vi "Log to Excel.vi"(8 "error in":errorcluster, 11 "tdms file in":refnum<k34>) -> (0 "error out":errorcluster, 2 "appended array":dbl[][][](array[numeric]), 3 "tdms file out":refnum<k34>)   [LabVIEW 2014, in "Logger.lvlib"]
uses:
  Logger.lvlib
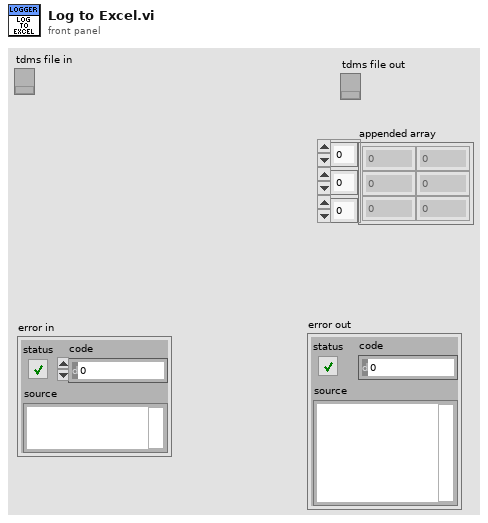
[diagram p1: front panel]
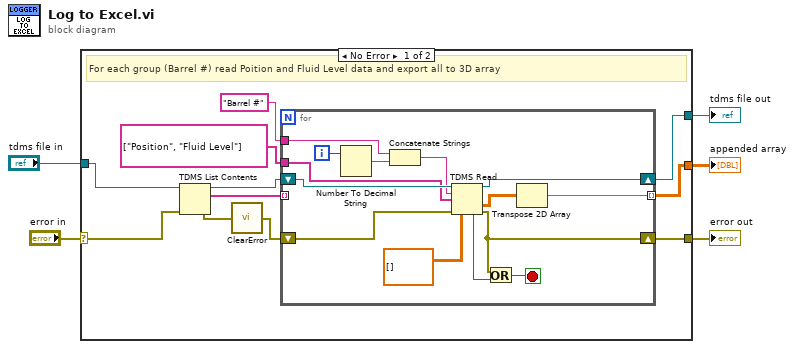
[diagram p0: block diagram]
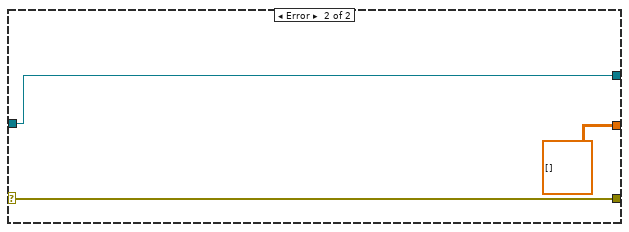
[diagram p2: hidden frame]
diagram:
  n1 = case shown="No Error" "error in" {
    selector: "error in" -> [w10 w33]
    tunnel: [w15 dbl[][][] []] -> w5
    tunnel: [w14 w33] -> w4
    tunnel: [w12 w32] -> w3
    tunnel: "tdms file in" -> [w7 w32]
    frame No Error {
      # "For each group (Barrel #) read Poition and Fluid Level data and export all to 3D array"
      n2 = TDMS List Contents(4:w10, 7:w7) -> (0:w6:errorcluster, 2:w11:string[], 3:w8:refnum<k34>)  [unwired: 1 in, 1 out]
      n3 = call <vilib>:"ClearError.vi"("error in (no error)"=w6) -> ("error out"=w9:errorcluster)
      n4 = for {
        tunnel: string[] ["Position", "Fluid Level"] -> [w22]
        tunnel: "Barrel #" -> [w27]
        tunnel: [w20] -> w15 mode=indexing
        shift-right: [w19] -> w14
        shift-left: w9 -> [w29]
        tunnel: w11 -> [_] mode=indexing
        shift-right: [w24] -> w12
        shift-left: w8 -> [w30]
        i -> [w25]
        stop <- w17 stop-if-true
        n5 = Number To Decimal String(number=w25) -> (decimal integer string=w26:string)  [unwired: 1 in]
        n6 = Concatenate Strings(w27, w26) -> (w23:string)
        n7 = TDMS Read(0:w30, 5:w23, 7:w22, 11:w29, 12:dbl[][] [] ("appended array")) -> (4:w24:refnum<k34>, 10:w21:dbl[][], 14:w18:bool, 15:w19:errorcluster)  [unwired: 3 in, 2 out]
        n8 = Or(x=w19, y=w18) -> (x .or. y?=w17:bool)
        n9 = Transpose 2D Array(2D array=w21) -> (transposed array=w20:dbl[][])
      }
    }
    frame Error {
    }
  }
  "error out" <- w4
  "appended array" <- w5
  "tdms file out" <- w3
